vi "Path To String.vi"(8 "error in (no error)":errorcluster, 10 "Path":path, 11 "Registry Object":refnum<class "Carya Config.lvclass">) -> (0 "error out":errorcluster, 2 "resulting string":string, 3 "Registry Object":refnum<class "Carya Config.lvclass">)   [LabVIEW 2013, in "Carya Config.lvclass"]
doc: "Copyright 2018, Carya Automatisering, Wiebe Walstra."
uses:
  Carya Config.lvclass
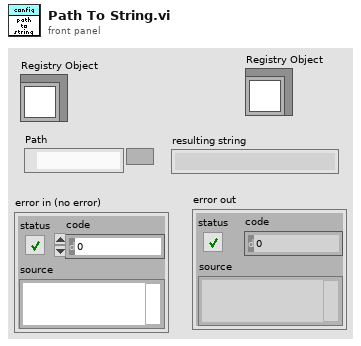
[diagram p1: front panel]
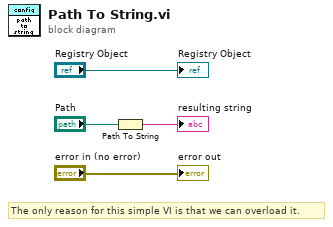
[diagram p0: block diagram]
diagram:
  # "The only reason for this simple VI is that we can overload it."
  n1 = Path To String(path="Path") -> (string=→"resulting string":string)
  "Registry Object" <- "Registry Object"
  "error out" <- "error in (no error)"
